vi "solar_write SOLARUIUnpin.vi"(8 "error in (no error)":errorcluster, 10 "Target":string, 11 "solar in":refnum<class "solar.lvclass">) -> (0 "error out":errorcluster, 3 "solar out":refnum<class "solar.lvclass">)   [LabVIEW 2018, in "solar.lvclass"]
doc: "This unpins (i.e. pops out) the target from the SOLAR user interface. Use the SOLAR.UI.Active to re-pin the target."
uses:
  solar.lvclass
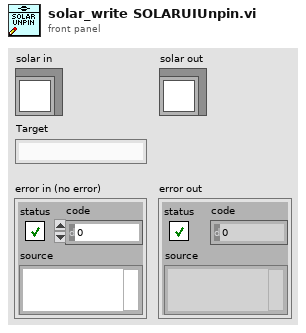
[diagram p1: front panel]
types:
  T1 = typedef "solar_ctl SOLAR Refnum.ctl" = refnum<k1>
  T2 = typedef "solar_ctl SOLAR Global.ctl" = cluster{"Targets":T3[], "AppDir":path, "solar.ini":path, "ConfigsDir":path, "CosmosDir":path, "LogsDir":path, "ExePath":path, "ExeVersion":string, "PartNum":string, "AppSetup":string, "Title":string, "Main.ini":path, "Temp.ini":path, "vSOLAR":string, "Splash.png":string, "SplashWait":i32, "SOLARUE":refnum<user-event>, "VoyagerRefnum":T4, "QTimerRefnum":T5}
  T3 = typedef "solar_ctl Target Global.ctl" = cluster{"Target":string, "Q":refnum<queue>, "UE":refnum<user-event>, "VI":refnum<vi>, "Menu":refnum<k9>, "Data":refnum<data-value>, "Attributes":variant}
  T4 = typedef "solar_voy_ctl Voyager Refnum.ctl" = refnum<k1>
  T5 = typedef "solar_qtimer_ctl Refnum.ctl" = refnum<k1>
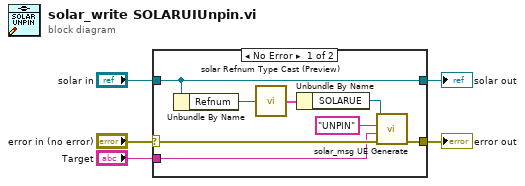
[diagram p0: block diagram]
diagram:
  n1 = case shown="No Error" "error in (no error)" {
    selector: "error in (no error)" -> [w9 w15]
    tunnel: "solar in" -> [w11 w14]
    tunnel: [w8 w15] -> w3
    tunnel: [w11 w14] -> w2
    tunnel: "Target" -> [w7 _]
    frame No Error {
      n2 = Unbundle By Name(w11) -> ("Refnum"=w13:T1)
      n3 = call "solar Refnum Type Cast (Preview).vi"("Refnum"=w13) -> ("SOLAR"=w12:T2)  [unwired: 8 in]
      n4 = Unbundle By Name(w12) -> ("SOLARUE"=w6:refnum<user-event>)
      n5 = call "solar_msg UE Generate.vi"("error in (no error)"=w9, "CMD_DATA (Last)"=w7, "CMD (Last)"="UNPIN" ("Packet"), "UserEvent in"=w6) -> ("error out"=w8:errorcluster)  [unwired: 6 in, 1 out]
    }
    frame Error {
    }
  }
  "error out" <- w3
  "solar out" <- w2
